vi "storePerm.vi"(0 "_Controller in":refnum<class "_Controller.lvclass">, 5 "error in (no error)":errorcluster) -> (14 "_Controller out":refnum<class "_Controller.lvclass">, 19 "error out":errorcluster)   [LabVIEW 2013, in "classes.lvlib" / "_Controller.lvclass"]
doc: "Stores the previously written parameters permanently to non-volatile memory.\n\nProduced By:\n\n<B>Kod Integrations, LLC</B>\n4835 Marianne Drive\nMount Airy, MD 21771\nhttp://www.kodintegrations.com\nemail: info@kodintegrations.com\nphone: (240) 687-1288"
uses:
  _Controller.lvclass
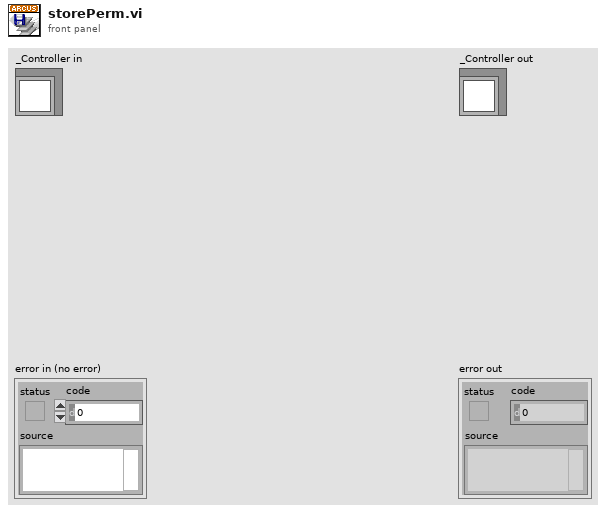
[diagram p1: front panel]
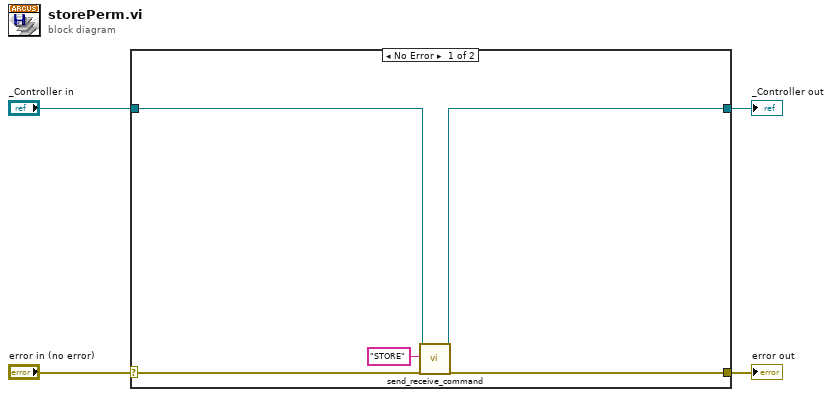
[diagram p0: block diagram]
diagram:
  n1 = case shown="No Error" "error in (no error)" {
    selector: "error in (no error)" -> [w9 w11]
    tunnel: [w8 w11] -> w3
    tunnel: [w6 w10] -> w1
    tunnel: "_Controller in" -> [w7 w10]
    frame No Error {
      n2 = call "send_receive_command.vi"("reference (in)"=w7, "ASCII Command (in)"="STORE", "error in (no error)"=w9) -> ("reference (out)"=w6:refnum<class "_Controller.lvclass">, "error out"=w8:errorcluster)  [unwired: 12 in, 3 out]
    }
    frame Error {
    }
  }
  "error out" <- w3
  "_Controller out" <- w1
